vi "FC_Test_Get_Comp_Attributes.vi"() -> ()   [LabVIEW 2013]
uses:
  FC_Competition Attributes.ctl
  FC_Target.ctl
  FC_FIRST Client.lvlib
panel:
  out "Comp Data Cluster":T1
  in  "Competition ID# (Ex: 7689)":string="7689"
  # "This VI demonstrates getting the attributes of a competition"
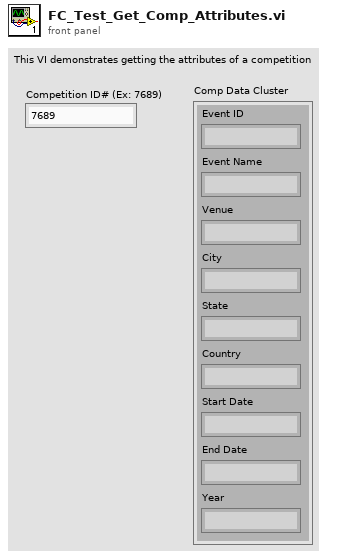
[diagram p1: front panel]
types:
  T1 = typedef "FC_FIRST Client.lvlib/FC_Competition Attributes.ctl" = cluster{"Event ID":string, "Event Name":string, "Venue":string, "City":string, "State":string, "Country":string, "Start Date":string, "End Date":string, "Year":string}
  T2 = typedef "FC_FIRST Client.lvlib/FC_Target.ctl" = enum16{"Teams", "Competitions"}
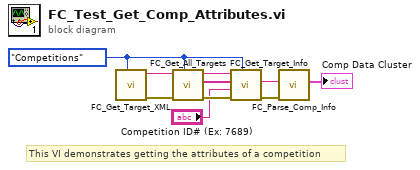
[diagram p0: block diagram]
diagram:
  w6 = FC_Target."Competitions" ("Enum")
  # "This VI demonstrates getting the attributes of a competition"
  n1 = call "FC_Get_Target_XML.vi"("Target"=w6) -> ("error out"=w7:errorcluster, "All Teams XML"=w10:string)  [unwired: 9 in]
  n2 = call "FC_Get_All_Targets.vi"("Target"=w6, "Error In"=w7, "Target XML"=w10) -> ("error out"=w8:errorcluster, "Array of Targets"=w5:string[], "Copy of Target XML"=w9:string)  [unwired: 6 in]
  n3 = call "FC_Get_Target_Info.vi"("Target"=w6, "Error In"=w8, "Desired Target"="Competition ID# (Ex: 7689)", "Array of Targets"=w5, "Target XML"=w9) -> ("error out"=w2:errorcluster, "Target Info"=w3:string)  [unwired: 5 in]
  n4 = call "FC_Parse_Comp_Info.vi"("Error In"=w2, "All Competition Data"=w3) -> ("Comp Data Cluster"=→"Comp Data Cluster":T1)  [unwired: 8 in, 1 out]
